vi "Results.Append Test Data to CSV Report File.vi"(6 "Remove Items":string[](array[string]), 8 "error in (no error)":errorcluster, 10 "Meas":T1[](array[typedef]) {"Status" items=["LOG", "PASS", "FAIL", "ERROR"]}, 11 "CSV File":path) -> (0 "error out":errorcluster, 2 "Appended":bool, 3 "Modified":bool)   [LabVIEW 2019]
uses:
  Result.Measurement Item.ctl
  Result.Measurement and Attribute Item Status.ctl
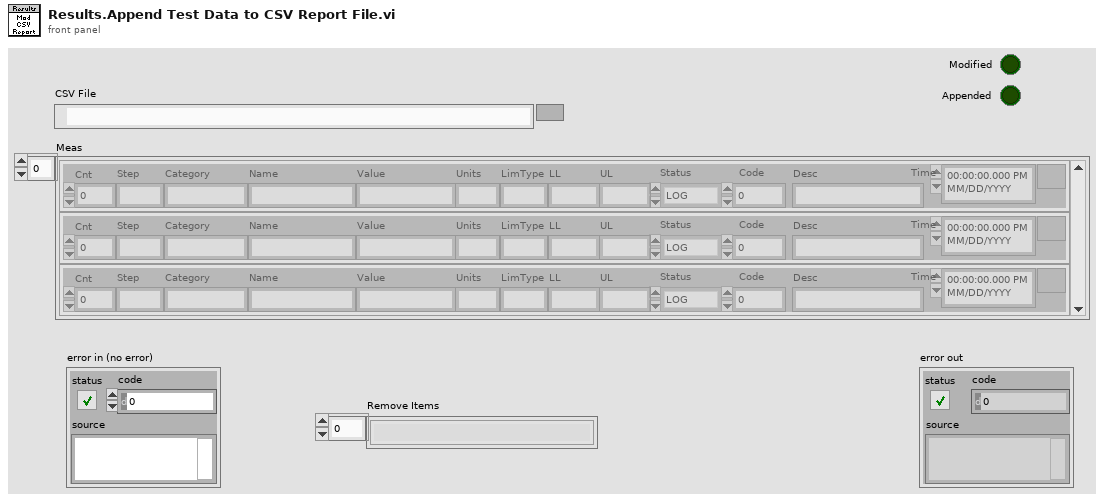
[diagram p1: front panel]
types:
  T1 = typedef "Result.Measurement Item.ctl" = cluster{"Cnt":i32, "Step":string, "Category":string, "Name":string, "Value":string, "Units":string, "LimType":string, "LL":string, "UL":string, "Status":T2, "Code":i32, "Desc":string, "Time":timestamp}
  T2 = typedef "Result.Measurement and Attribute Item Status.ctl" = i32
  T3 = enum16{"open", "replace", "create", "open or create", "replace or create", "replace or create with confirmation"}
  T4 = cluster{"NewRecords":string[][], "Data":string[], "Modified":bool, "Appended":bool, "CSV File":path}
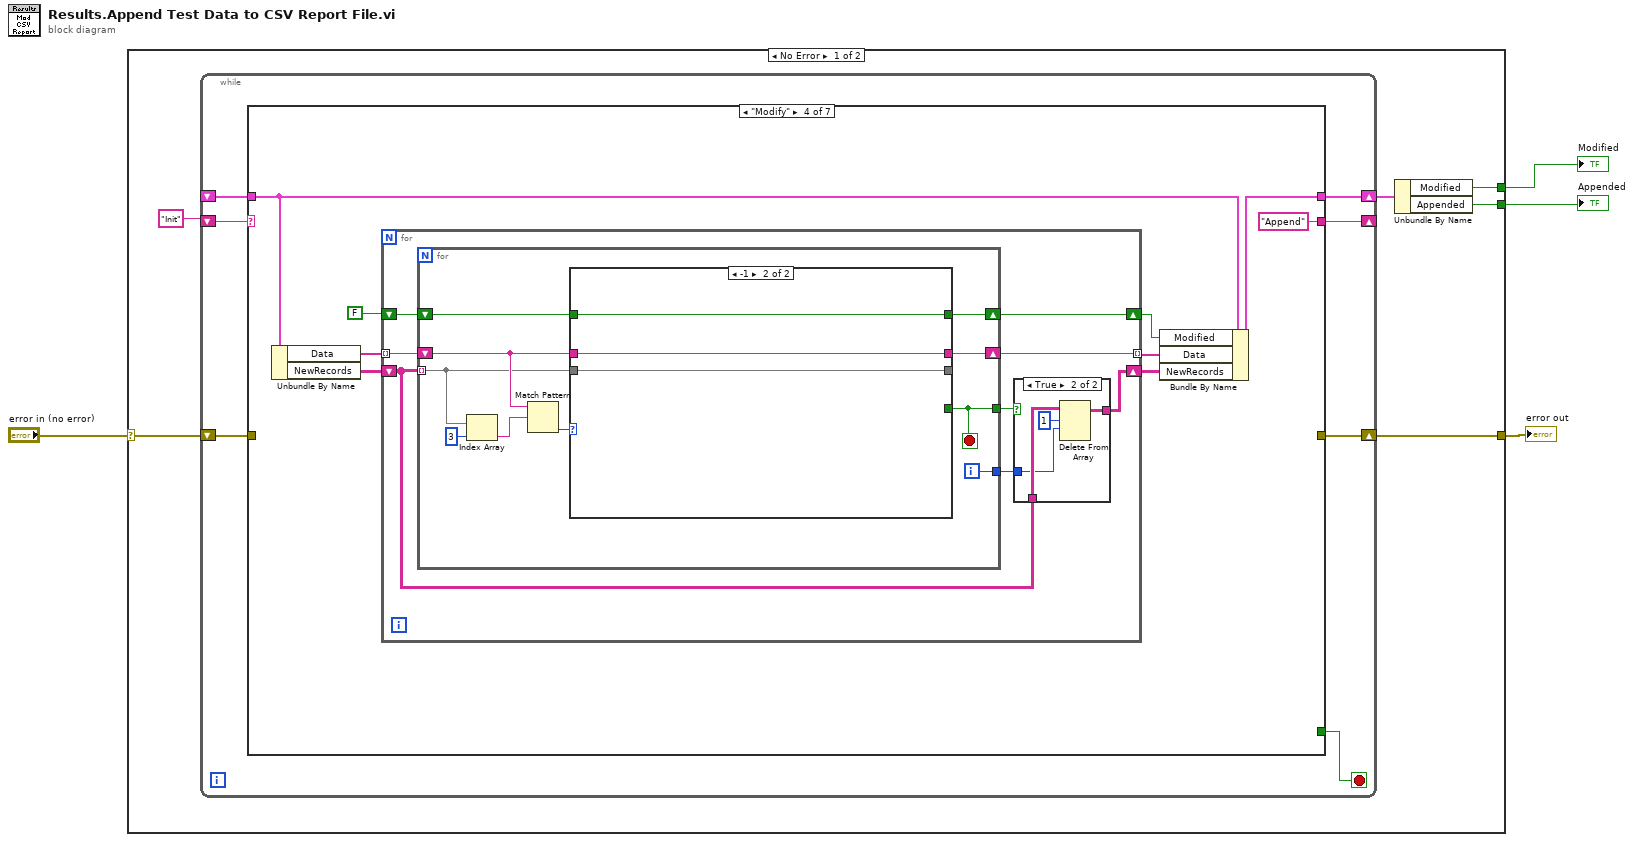
[diagram p0: block diagram]
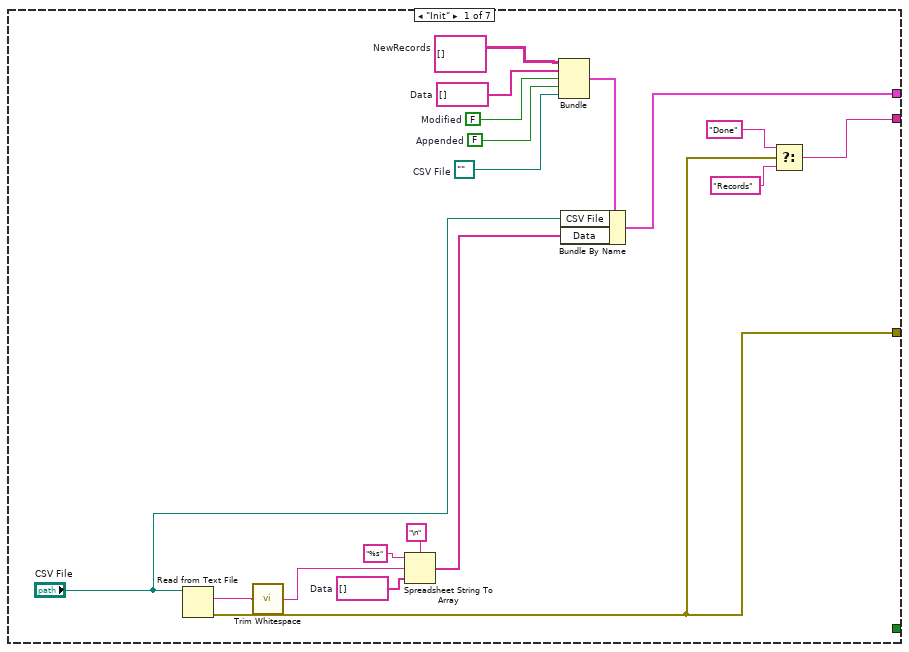
[diagram p2: hidden frame]
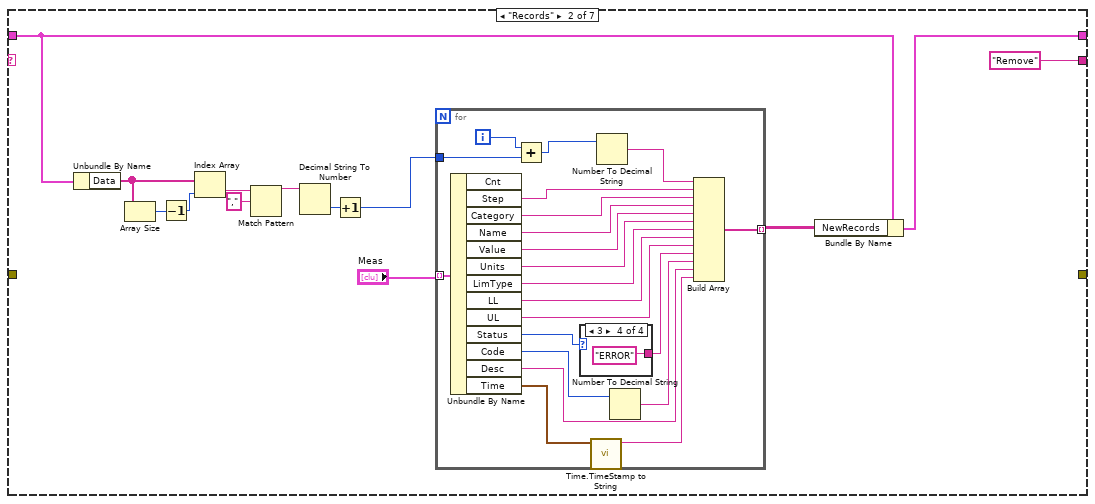
[diagram p3: hidden frame]
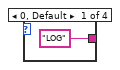
[diagram p4: hidden frame]
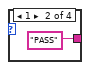
[diagram p5: hidden frame]
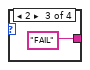
[diagram p6: hidden frame]
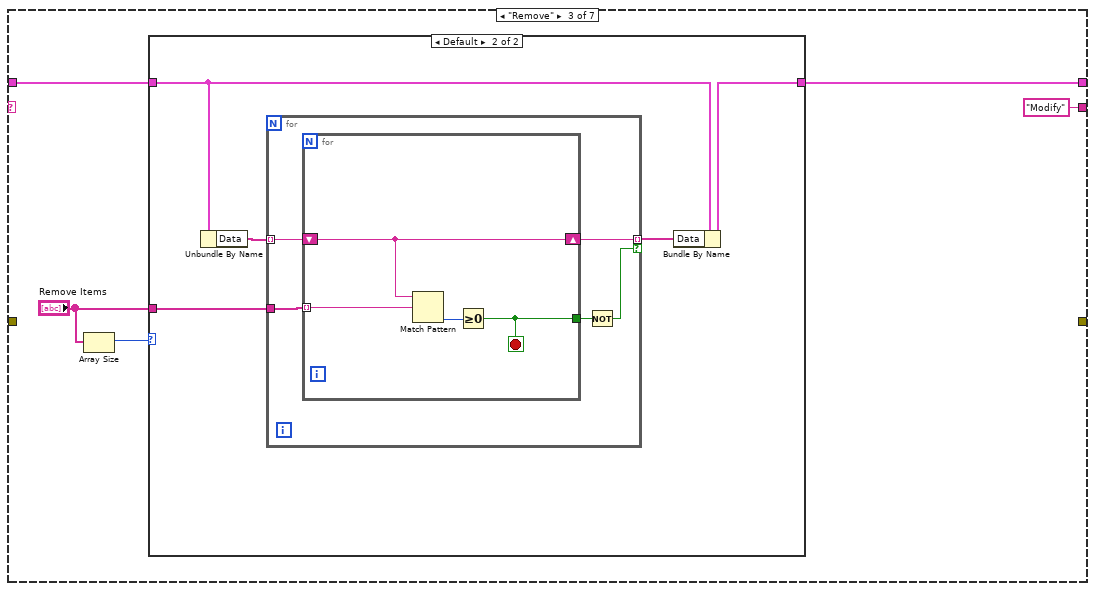
[diagram p7: hidden frame]
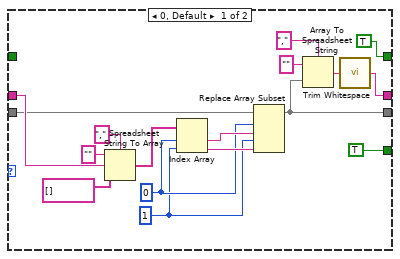
[diagram p10: hidden frame]
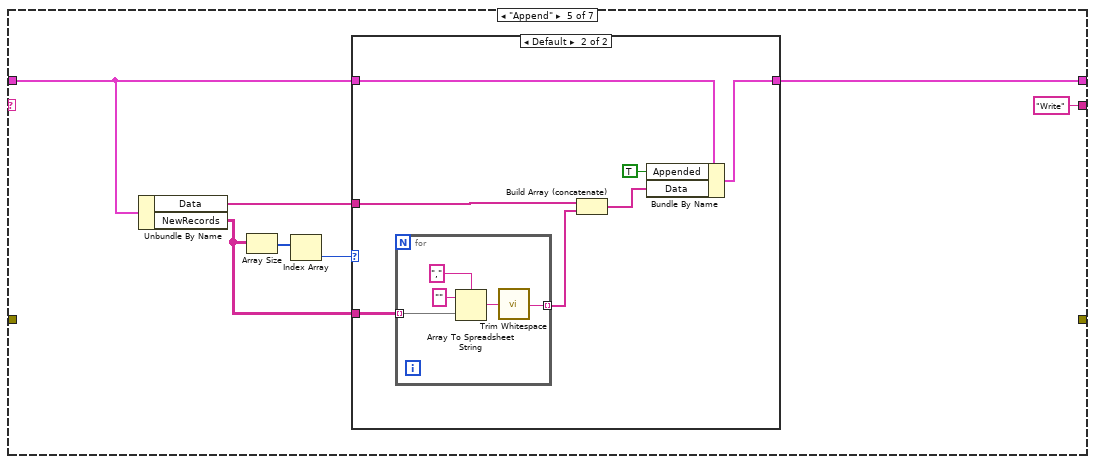
[diagram p11: hidden frame]
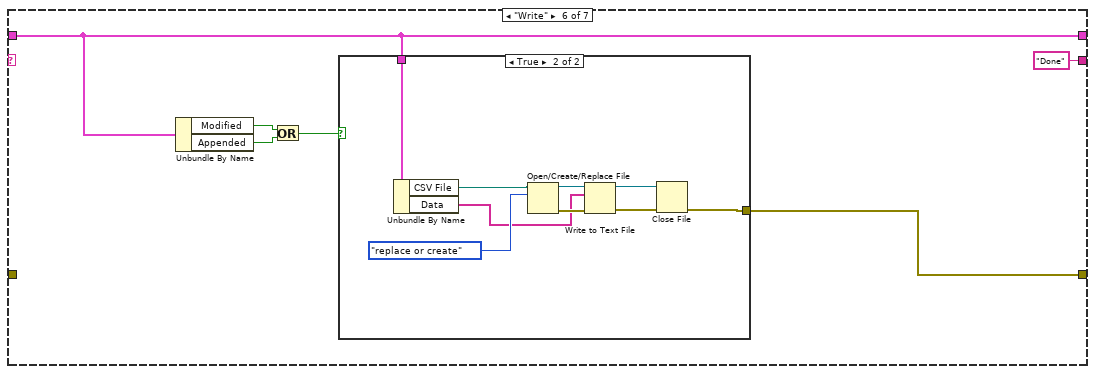
[diagram p13: hidden frame]
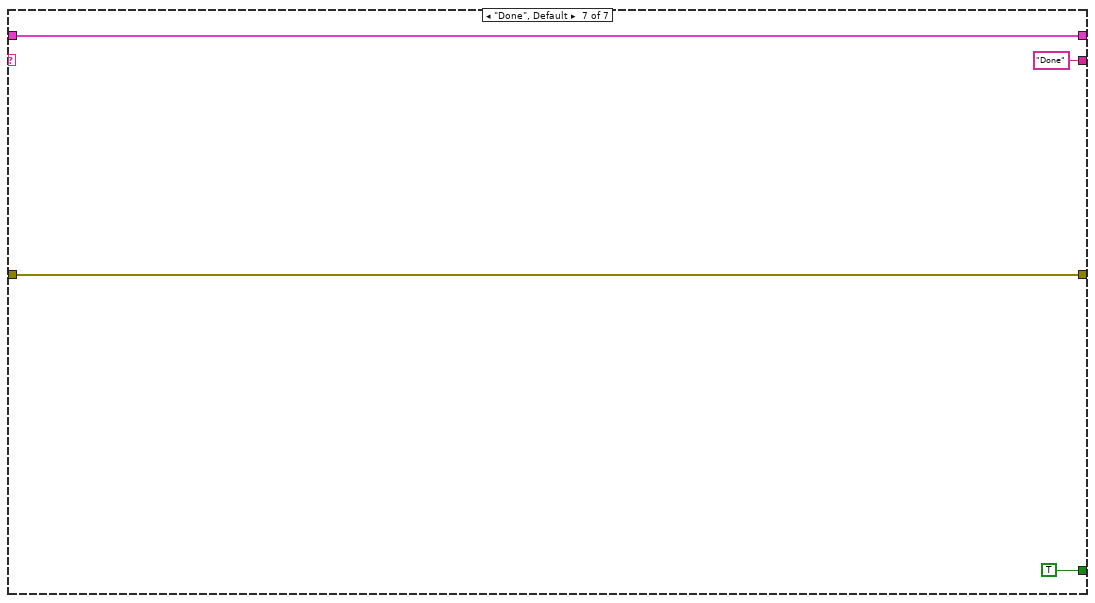
[diagram p15: hidden frame]
diagram:
  n1 = case shown="No Error" "error in (no error)" {
    selector: "error in (no error)" -> [w5 w184]
    tunnel: [w8 _] -> w4
    tunnel: [w7 _] -> w3
    tunnel: [w6 w184] -> w1
    frame No Error {
      n2 = while {
        shift-right: [w15] -> _
        shift-left: "Init" -> [w17]
        shift-right: [w16] -> w9
        shift-left: _ -> [w13]
        shift-right: [w12] -> w6
        shift-left: w5 -> [w11]
        stop <- w14 stop-if-true
        n3 = case shown="\"Modify\"" w17 {
          tunnel: [w33 w45 w76 w95 w145 w167 w180] -> w16
          tunnel: [w28 "Remove" "Modify" "Append" "Write" "Done" "Done"] -> w15
          tunnel: [_ _ _ _ _ _ TRUE] -> w14
          tunnel: w13 -> [_ w44 w77 w98 w148 w167 w180]
          tunnel: [w20 _ _ _ _ w165 w181] -> w12
          tunnel: w11 -> [_ _ _ _ _ _ w181]
          frame "Init" {
            w19 = path ""  # CSV File
            w24 = string[][] []  # NewRecords
            w27 = string[] []  # Data
            w31 = FALSE  # Appended
            w32 = FALSE  # Modified
            w35 = string[] []  # Data
            n4 = Read from Text File(file (use dialog)="CSV File") -> (text=w22:string, error out=w20:errorcluster)  [unwired: 3 in, 2 out]
            n5 = call <vilib>:"Trim Whitespace.vi"("string"=w22) -> ("trimmed string"=w21:string)  [unwired: 1 in]
            n6 = Spreadsheet String To Array(delimiter (Tab)="\n", format string="%s", spreadsheet string=w21, array type (2D Dbl)=w27) -> (array=w23:string[])
            n7 = Bundle("NewRecords"=w24, "Data"=w35, "Modified"=w32, "Appended"=w31, "CSV File"=w19) -> (w34:T4)  [unwired: 1 in]
            n8 = Bundle By Name(cluster=w34, "CSV File"="CSV File", "Data"=w23) -> (w33:T4)
            n9 = Select(t="Done", s=w20, f="Records") -> (s? t:f=w28:string)
          }
          frame "Records" {
            n10 = Unbundle By Name(w44) -> ("Data"=w41:string[])
            n11 = Array Size(array=w41) -> (size(s)=w43:i32)
            n12 = Decrement(x=w43) -> (x-1=w42:i32)
            n13 = Index Array(array=w41, index=w42) -> (element=w40:string)
            n14 = Match Pattern(string=w40, regular expression=",") -> (before substring=w38:string)  [unwired: 1 in, 3 out]
            n15 = Decimal String To Number(string=w38) -> (number=w37:i32)  [unwired: 2 in, 1 out]
            n16 = Increment(x=w37) -> (x+1=w36:i32)
            n17 = for {
              tunnel: "Meas" -> [w69] mode=indexing
              tunnel: [w57] -> w46 mode=indexing
              tunnel: w36 -> [w49]
              i -> [w50]
              n18 = Unbundle By Name(w69) -> ("Step"=w51:string, "Category"=w67:string, "Name"=w66:string, "Value"=w65:string, "Units"=w64:string, "LimType"=w63:string, "LL"=w62:string, "UL"=w61:string, "Status"=w56:T2, "Code"=w60:i32, "Desc"=w58:string, "Time"=w54:timestamp)  [unwired: 1 out]
              n19 = Add(x=w50, y=w49) -> (x+y=w52:i32)
              n20 = case shown="3" w56 {
                tunnel: ["LOG" "PASS" "FAIL" "ERROR"] -> w55
                frame 0, Default {
                }
                frame 1 {
                }
                frame 2 {
                }
                frame 3 {
                }
              }
              n21 = call "Time.TimeStamp to String.vi"("Time Stamp in"=w54) -> ("Time String Out"=w53:string)  [unwired: 10 in]
              n22 = Number To Decimal String(number=w52) -> (decimal integer string=w68:string)  [unwired: 1 in]
              n23 = Number To Decimal String(number=w60) -> (decimal integer string=w59:string)  [unwired: 1 in]
              n24 = Build Array(w68, w51, w67, w66, w65, w64, w63, w62, w61, w55, w59, w58, w53) -> (w57:string[])
            }
            n25 = Bundle By Name(cluster=w44, "NewRecords"=w46) -> (w45:T4)
          }
          frame "Remove" {
            n26 = Array Size(array="Remove Items") -> (size(s)=w74:i32)
            n27 = case shown="Default" w74 {
              tunnel: w77 -> [w79 w83]
              tunnel: [w79 w82] -> w76
              tunnel: "Remove Items" -> [_ w80]
              frame 0 {
              }
              frame Default {
                n28 = Unbundle By Name(w83) -> ("Data"=w84:string[])
                n29 = for {
                  tunnel: w84 -> [w89] mode=indexing
                  tunnel: [w88] -> w81 mode=indexing if=w85
                  tunnel: w80 -> [w87]
                  n30 = for {
                    tunnel: w87 -> [w93] mode=indexing
                    shift-right: [w92] -> w88
                    shift-left: w89 -> [w92]
                    tunnel: [w90] -> w86
                    stop <- w90 stop-if-true
                    n31 = Match Pattern(string=w92, regular expression=w93) -> (offset past match=w91:i32)  [unwired: 1 in, 3 out]
                    n32 = Greater Or Equal To 0?(x=w91) -> (x >= 0?=w90:bool)
                  }
                  n33 = Not(x=w86) -> (.not. x?=w85:bool)
                }
                n34 = Bundle By Name(cluster=w83, "Data"=w81) -> (w82:T4)
              }
            }
          }
          frame "Modify" {
            n35 = Unbundle By Name(w98) -> ("Data"=w101:string[], "NewRecords"=w100:string[][])
            n36 = for {
              tunnel: w101 -> [w110] mode=indexing
              shift-right: [w108] -> w97
              shift-left: FALSE -> [w109]
              shift-right: [w104] -> w96
              shift-left: w100 -> [w106]
              tunnel: [w107] -> w94 mode=indexing
              n37 = for {
                tunnel: w106 -> [w121] mode=indexing
                shift-right: [w118] -> w108
                shift-left: w109 -> [w119]
                tunnel: [w117] -> w103
                tunnel: [w116] -> w105
                shift-right: [w120] -> w107
                shift-left: w110 -> [w122]
                i -> [w116]
                stop <- w117 stop-if-true
                n38 = Index Array(array=w121, index=3) -> (element=w124:string)
                n39 = Match Pattern(string=w122, regular expression=w124) -> (offset past match=w123:i32)  [unwired: 1 in, 3 out]
                n40 = case shown="-1" w123 {
                  tunnel: w122 -> [w136 w144]
                  tunnel: w121 -> [w132 w142]
                  tunnel: [w138 w144] -> w120
                  tunnel: w119 -> [_ w143]
                  tunnel: [TRUE w143] -> w118
                  tunnel: [w132 w142] -> _
                  tunnel: [TRUE _] -> w117
                  frame 0, Default {
                    w127 = 1 ("index")
                    w128 = 0 ("index")
                    n41 = Spreadsheet String To Array(delimiter (Tab)=",", format string="", spreadsheet string=w136, array type (2D Dbl)=string[] [] ("format string")) -> (array=w131:string[])
                    n42 = Index Array(array=w131, index #1=w128, index #2=w127) -> (element #1=w130:string, element #2=w129:string)
                    n43 = Replace Array Subset(array=w132, new element #1=w130, index #1=w128, new element #2=w129, index #2=w127) -> ()  [unwired: 1 out]
                    n44 = Array To Spreadsheet String(delimiter (Tab)=",", array=w132, 3:"" ("format string")) -> (spreadsheet string=w139:string)
                    n45 = call <vilib>:"Trim Whitespace.vi"("string"=w139) -> ("trimmed string"=w138:string)  [unwired: 1 in]
                  }
                  frame -1 {
                  }
                }
              }
              n46 = case shown="True" w103 {
                tunnel: w106 -> [w111 w115]
                tunnel: w105 -> [_ w113]
                tunnel: [w111 w112] -> w104
                frame False {
                }
                frame True {
                  n47 = Delete From Array(array=w115, length=1, index (row)=w113) -> (array with subset deleted=w112:string[][])  [unwired: 1 in, 1 out]
                }
              }
            }
            n48 = Bundle By Name(cluster=w98, "Modified"=w97, "Data"=w94, "NewRecords"=w96) -> (w95:T4)
          }
          frame "Append" {
            n49 = Unbundle By Name(w148) -> ("Data"=w150:string[], "NewRecords"=w149:string[][])
            n50 = Array Size(array=w149) -> (size(s)=w147:i32[])
            n51 = Index Array(array=w147) -> (element=w146:i32)  [unwired: 1 in]
            n52 = case shown="Default" w146 {
              tunnel: w150 -> [_ w156]
              tunnel: w149 -> [_ w154]
              tunnel: [w152 w159] -> w145
              tunnel: w148 -> [w152 w158]
              frame 0 {
              }
              frame Default {
                n53 = for {
                  tunnel: [w161] -> w155 mode=indexing
                  tunnel: w154 -> [w162] mode=indexing
                  n54 = Array To Spreadsheet String(delimiter (Tab)=",", array=w162, 3:"" ("format string")) -> (spreadsheet string=w160:string)
                  n55 = call <vilib>:"Trim Whitespace.vi"("string"=w160) -> ("trimmed string"=w161:string)  [unwired: 1 in]
                }
                n56 = Build Array (concatenate)(w156, w155) -> (w153:string[])
                n57 = Bundle By Name(cluster=w158, "Appended"=TRUE, "Data"=w153) -> (w159:T4)
              }
            }
          }
          frame "Write" {
            n58 = Unbundle By Name(w167) -> ("Modified"=w170:bool, "Appended"=w169:bool)
            n59 = Or(x=w170, y=w169) -> (x .or. y?=w168:bool)
            n60 = case shown="True" w168 {
              tunnel: w167 -> [_ w179]
              tunnel: [_ w171] -> w165
              frame False {
              }
              frame True {
                n61 = Unbundle By Name(w179) -> ("CSV File"=w177:path, "Data"=w175:string[])
                n62 = Open/Create/Replace File(file path (use dialog)=w177, operation (0:open)=T3."replace or create") -> (refnum out=w174:refnum<file>, error out=w178:errorcluster)  [unwired: 4 in, 1 out]
                n63 = Write to Text File(file (use dialog)=w174, text=w175, error in=w178) -> (refnum out=w173:refnum<file>, error out=w172:errorcluster)  [unwired: 1 in, 1 out]
                n64 = Close File(refnum=w173, error in=w172) -> (error out=w171:errorcluster)  [unwired: 1 out]
              }
            }
          }
          frame "Done", Default {
          }
        }
      }
      n65 = Unbundle By Name(w9) -> ("Modified"=w8:bool, "Appended"=w7:bool)
    }
    frame Error {
    }
  }
  "Modified" <- w4
  "Appended" <- w3
  "error out" <- w1
